vi "OA Add Mode.vi"(7 "uiModeDescriptionLen":u32, 8 "error in (no error)":errorcluster, 9 "pcModeDescription":string, 10 "uiModeNameLen":u32, 11 "pcModeName":string) -> (0 "error out":errorcluster, 1 "pcModeDescription out":string, 2 "function return":u32, 3 "pcModeName out":string)   [LabVIEW 2014, in "atmcd32d.lvlib"]
doc: "unsigned int WINAPI OA_AddMode(char * pcModeName, unsigned int uiModeNameLen, char * pcModeDescription, unsigned int uiModeDescriptionLen);"
uses:
  atmcd32d.lvlib
  atmcd32d.dll
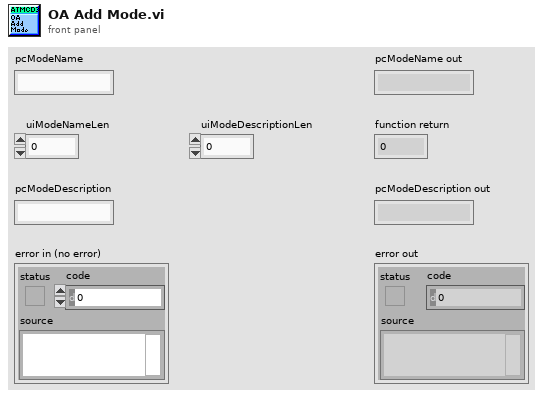
[diagram p1: front panel]
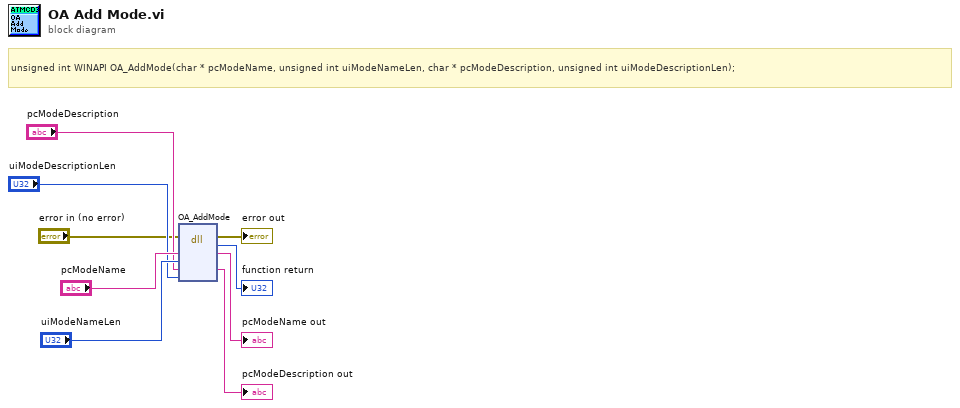
[diagram p0: block diagram]
diagram:
  # "unsigned int WINAPI OA_AddMode(char * pcModeName, unsigned int uiModeNameLen, char * pcModeDescription, unsigned int uiModeDescriptionLen);"
  n1 = dll-call lib="C:/Users/Bakir/Documents/Lambda2-Testing/lib/Andorlib/atmcd32d.*" fn="OA_AddMode"(error in="error in (no error)", "pcModeName"="pcModeName", "uiModeNameLen"="uiModeNameLen", "pcModeDescription"="pcModeDescription", "uiModeDescriptionLen"="uiModeDescriptionLen") -> (error out=→"error out":errorcluster, →"function return":u32, "pcModeName"=→"pcModeName out":string, "pcModeDescription"=→"pcModeDescription out":string)  [unwired: 4 in, 1 out]
